vi "温度测试.vi"() -> ()   [LabVIEW 2010]
uses:
  Instance           5 16Saved   温度测试 .vi
  Instance           2 16Saved   温度测试 .vi
  Instance           4 16Saved   温度测试 .vi
  Instance           3 16Saved   温度测试 .vi
  Instance           1 16Saved   温度测试 .vi
  <vilib>/Analysis/NI_AALBase.lvlib
panel:
  out "波形图表":cluster{"Y":dbl, dbl}(graph)
  out "热电阻电压（mV）":dbl format="%#_4g"
  out "热敏电阻电压（mV）":dbl format="%_3g"
  out "温度（℃）":dbl(slide) scale=0.0..100.0
  in  "停止":bool
  # "温度测试实验"
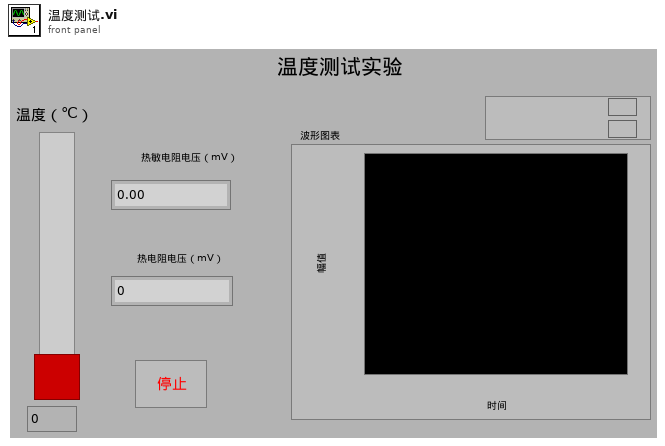
[diagram p1: front panel]
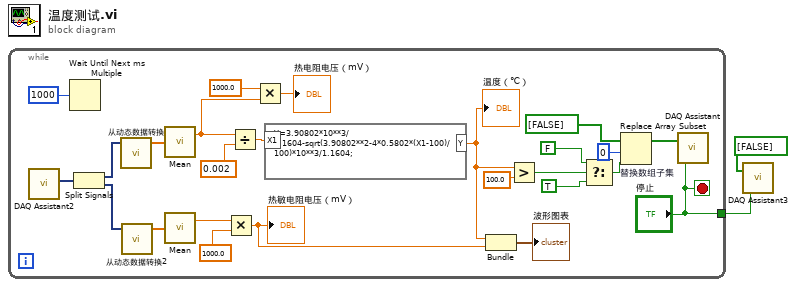
[diagram p0: block diagram]
diagram:
  n1 = while {
    tunnel: ["停止"] -> w1
    stop <- "停止" stop-if-true
    n2 = call "DAQ Assistant2"() -> ("data"=w18:dynamicdata)  [unwired: 16 in, 3 out]
    n3 = Wait Until Next ms Multiple(millisecond multiple=u32 1000 ("毫秒倍数")) -> ()  [unwired: 1 out]
    n4 = Split Signals(w18) -> (w17:dynamicdata, w14:dynamicdata)  [unwired: 2 in]
    n5 = call "从动态数据转换"("Dynamic Data Type"=w17) -> ("Array"=w16:dbl[])  [unwired: 3 in]
    n6 = call "从动态数据转换2"("Dynamic Data Type"=w14) -> ("Array"=w15:dbl[])  [unwired: 3 in]
    n7 = call <vilib>:"Mean.vi"("X"=w16) -> ("mean"=w7:dbl)  [unwired: 1 out]
    n8 = call <vilib>:"Mean.vi"("X"=w15) -> ("mean"=w10:dbl)  [unwired: 1 out]
    n9 = Multiply(x=w10, y=1000.0) -> (x*y=w4:dbl)
    "热敏电阻电压（mV）" <- w4
    n10 = Divide(x=w7, y=0.002) -> (x/y=w13:dbl)
    n11 = Multiply(x=1000.0 ("y"), y=w7) -> (x*y=→"热电阻电压（mV）":dbl)
    n12 = formula code="Y=3.90802*10**3/1.1604-sqrt(3.90802**2-4*0.5802*(X1-100)/100)*10**3/1.1604;"("X1"=w13) -> ("Y"=w5:dbl)
    "温度（℃）" <- w5
    n13 = Bundle("Y"=w5, w4) -> (→"波形图表":cluster{"Y":dbl, dbl})  [unwired: 1 in]
    n14 = Greater?(x=w5, y=100.0) -> (0:w23:bool)
    n15 = Select(t=FALSE, s=w23, f=TRUE) -> (s? t:f=w21:bool)
    n16 = Replace Array Subset "替换数组子集"(array=bool[] [FALSE] ("data"), new element=w21, index=0 ("索引")) -> (w22:bool[])
    n17 = call "DAQ Assistant"("data"=w22, "stop (T)"="停止") -> ()  [unwired: 16 in, 2 out]
  }
  n18 = call "DAQ Assistant3"("data"=bool[] [FALSE], "stop (T)"=w1) -> ()  [unwired: 16 in, 2 out]
